vi "PowerSupplyMain.vi"() -> ()   [LabVIEW 2020]
uses:
  PowerSupply/PowerSupply.lvclass
  PowerSupply/PowerSupplyChannelSelection.ctl
panel:
  in  "Stop Button":bool
  out "error out":errorcluster
  in  "error in (no error)":errorcluster
  in  "Master Enable":bool
  in  "Enable Negative Supply":bool
  in  "Enable Positive Supply":bool
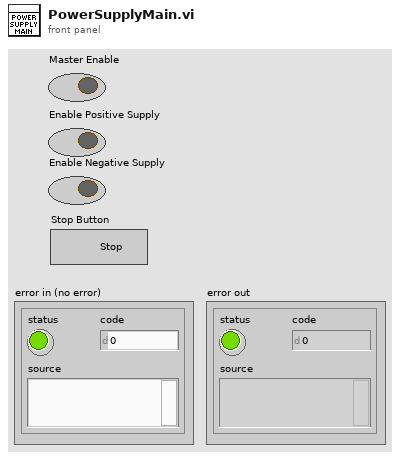
[diagram p1: front panel]
types:
  T1 = typedef "PowerSupplyChannelSelection.ctl" = enum16{"ps/+5V", "ps/-5V"}
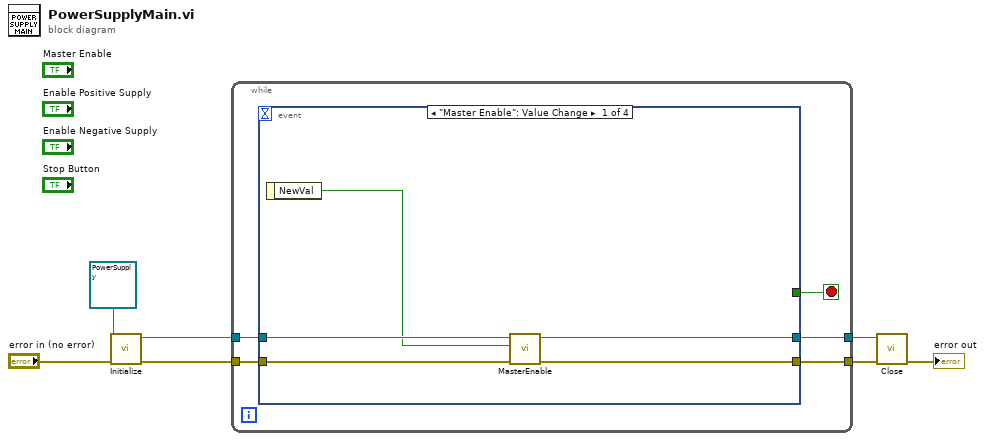
[diagram p0: block diagram]
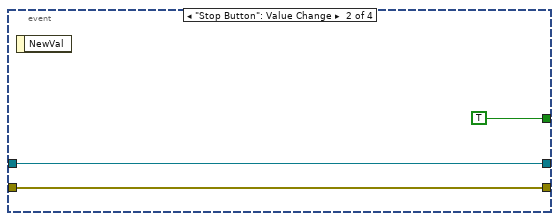
[diagram p2: hidden frame]
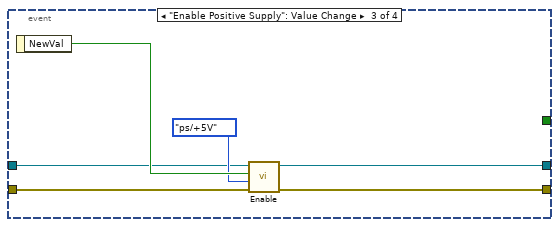
[diagram p3: hidden frame]
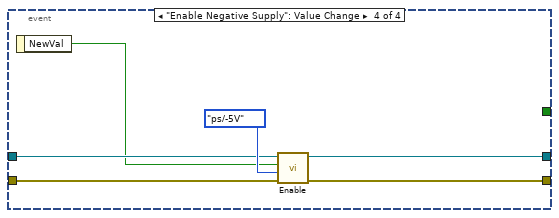
[diagram p4: hidden frame]
diagram:
  n1 = call-dynamic "Initialize.vi"("error in (no error)"="error in (no error)", "PowerSupply in"=refnum<class "PowerSupply.lvclass"> refnum) -> ("error out"=w6:errorcluster, "PowerSupply out"=w4:refnum<class "PowerSupply.lvclass">)  [unwired: 8 in]
  n2 = while {
    tunnel: w6 -> [w12]
    tunnel: w4 -> [w11]
    tunnel: [w10] -> w2
    tunnel: [w9] -> w3
    stop <- w8 stop-if-true
    n3 = event shown="[0] \"Master Enable\": Value Change" {
      selector: _ -> [_ _ _ _]
      dyn-events: _ -> [_ _ _ _]
      timeout: _ -> [_ _ _ _]
      tunnel: w12 -> [w17 w18 w26 w31]
      tunnel: [w16 w18 w25 w28] -> w10
      tunnel: w11 -> [w15 w19 w22 w30]
      tunnel: [w14 w19 w21 w29] -> w9
      tunnel: [_ TRUE _ _] -> w8
      event "Master Enable": Value Change {
        n4 = event-data() -> ("NewVal"=w13:bool)  [unwired: 1 in]
        n5 = call "MasterEnable.vi"("error in (no error)"=w17, "Master Enable"=w13, "PowerSupply in"=w15) -> ("error out"=w16:errorcluster, "PowerSupply out"=w14:refnum<class "PowerSupply.lvclass">)  [unwired: 7 in]
      }
      event "Stop Button": Value Change {
        n6 = event-data() -> ()  [unwired: 1 in, 1 out]
      }
      event "Enable Positive Supply": Value Change {
        n7 = event-data() -> ("NewVal"=w24:bool)  [unwired: 1 in]
        n8 = call "Enable.vi"("error in (no error)"=w26, "ChannelSelection"=PowerSupplyChannelSelection."ps/+5V", "Enable"=w24, "PowerSupply in"=w22) -> ("error out"=w25:errorcluster, "PowerSupply out"=w21:refnum<class "PowerSupply.lvclass">)  [unwired: 6 in]
      }
      event "Enable Negative Supply": Value Change {
        n9 = event-data() -> ("NewVal"=w27:bool)  [unwired: 1 in]
        n10 = call "Enable.vi"("error in (no error)"=w31, "ChannelSelection"=PowerSupplyChannelSelection."ps/-5V", "Enable"=w27, "PowerSupply in"=w30) -> ("error out"=w28:errorcluster, "PowerSupply out"=w29:refnum<class "PowerSupply.lvclass">)  [unwired: 6 in]
      }
    }
  }
  n11 = call-dynamic "Close.vi"("error in (no error)"=w2, "PowerSupply in"=w3) -> ("error out"=→"error out":errorcluster)  [unwired: 8 in, 1 out]
